vi "TotalConvTime.vi"(11 "fclk":dbl) -> (3 "TotalConvTime":dbl)   [LabVIEW 2021]
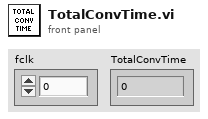
[diagram p1: front panel]
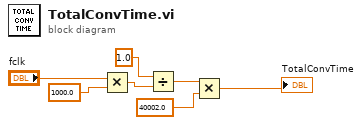
[diagram p0: block diagram]
diagram:
  n1 = Multiply(x="fclk", y=1000.0) -> (x*y=w4:dbl)
  n2 = Divide(x=1.0, y=w4) -> (x/y=w3:dbl)
  n3 = Multiply(x=w3, y=40002.0) -> (x*y=→"TotalConvTime":dbl)
